vi "Write Parameters.vi"(8 "error in (no error)":errorcluster, 10 "Parameters":T1={"Target Height"=0.0, "Elevator State Loop (ms)"=20, "Up Rate (Percentage)"=1.0, "Down Rate (Percentage)"=-1.0}, 11 "EL-Go To Height in":refnum<class "EL-Go To Height.lvclass">) -> (0 "error out":errorcluster, 3 "EL-Go To Height out":refnum<class "EL-Go To Height.lvclass">)   [LabVIEW 2014, in "Elevator.lvlib" / "EL-Go To Height.lvlib" / "EL-Go To Height.lvclass"]
uses:
  EL-Go To Height.lvclass
  Parameters.ctl
  EL-Go To Height.lvclass/EL-Go To Height.ctl
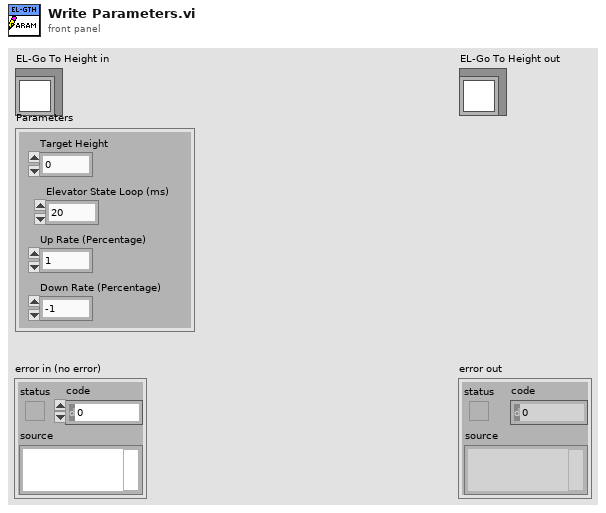
[diagram p1: front panel]
types:
  T1 = typedef "Elevator.lvlib/EL-Go To Height.lvlib/EL-Go To Height.lvclass/Parameters.ctl" = cluster{"Target Height":dbl, "Elevator State Loop (ms)":u32, "Up Rate (Percentage)":dbl, "Down Rate (Percentage)":dbl}
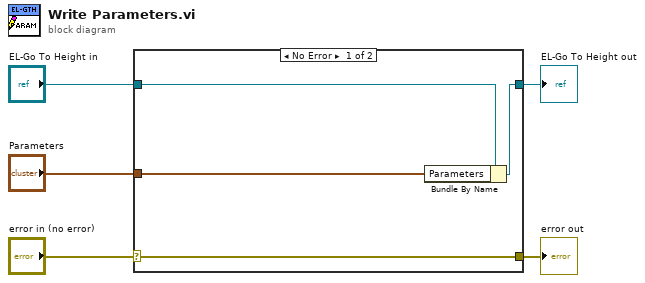
[diagram p0: block diagram]
diagram:
  n1 = case shown="No Error" "error in (no error)" {
    selector: "error in (no error)" -> [w9 w10]
    tunnel: [w9 w10] -> w4
    tunnel: [w7 w11] -> w2
    tunnel: "EL-Go To Height in" -> [w8 w11]
    tunnel: "Parameters" -> [w6 _]
    frame No Error {
      n2 = Bundle By Name(cluster=w8, "Parameters"=w6) -> (w7:refnum<class "EL-Go To Height.lvclass">)
    }
    frame Error {
    }
  }
  "error out" <- w4
  "EL-Go To Height out" <- w2
